vi "8.6-Crossbow Test.vi"() -> ()   [LabVIEW 2010]
uses:
  <vilib>/Instr/_visa.llb/VISA Configure Serial Port (Instr).vi
panel:
  in  "Array of Data to Send":u8[](array[numeric]) format="%.0x"
  in  "Use Checksum":bool
  out "error out":errorcluster
  out "Bytes at Port":u32
  in  "Stop Program":bool
  in  "baud rate (9600)":u32=38400
  in  "data bits (8)":u16=8
  in  "stop bits (10: 1 bit)":u16(ring)=10 items=["1.0"=10, "1.5"=15, "2.0"=20]
  in  "parity (0:none)":enum16{"None", "Odd", "Even", "Mark", "Space"}(ring)
  in  "Reset Port":bool
  in  "End Test":bool
  in  "VISA resource name":refnum<visa-resource-name>
  in  "Send String":bool
  out "Serial Port Output":string
  in  "String to write":string
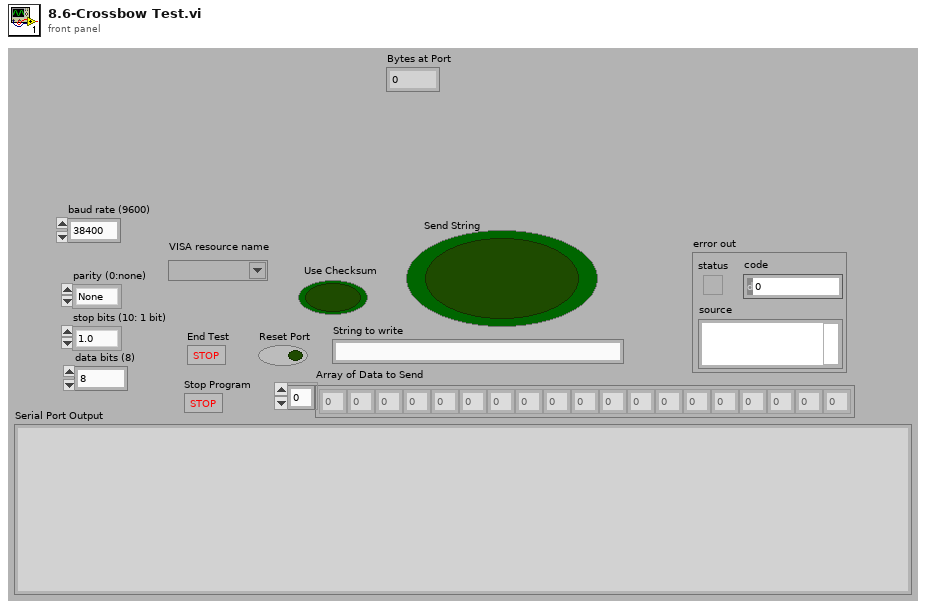
[diagram p1: front panel]
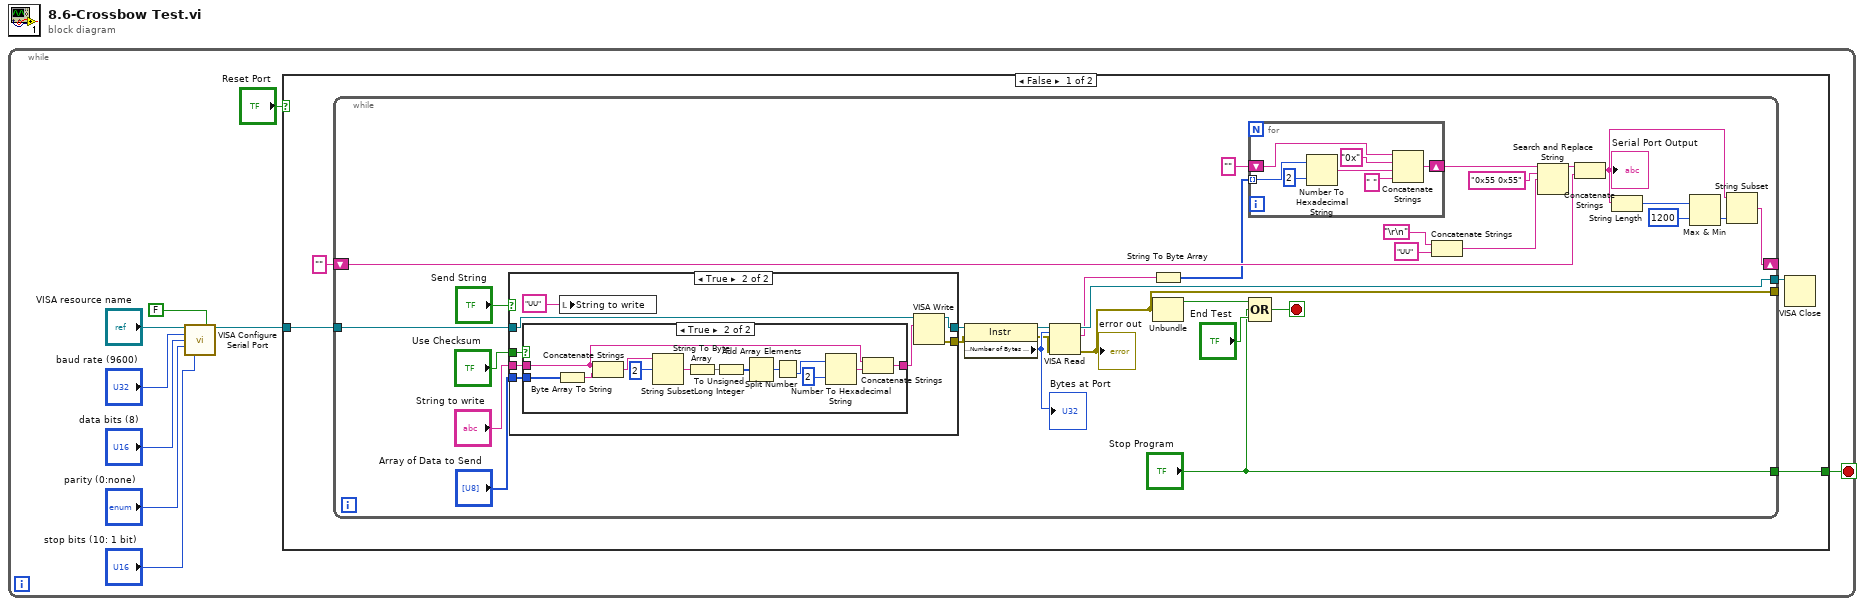
[diagram p0: block diagram]
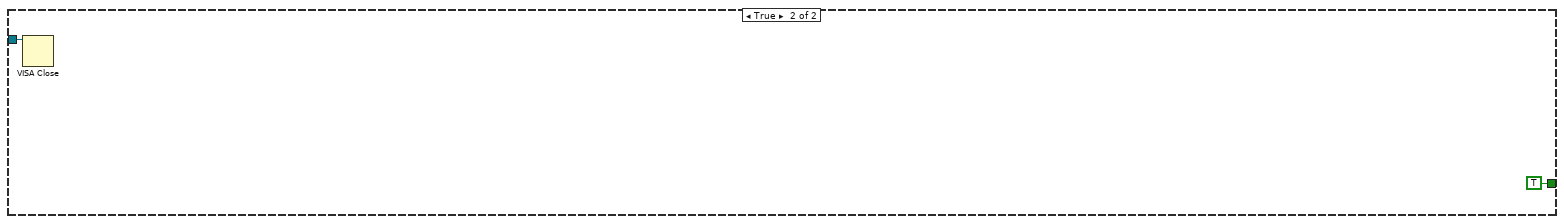
[diagram p4: hidden frame]
diagram:
  n1 = while {
    stop <- w1 stop-if-true
    n2 = call-poly "VISA Configure Serial Port"("VISA resource name"="VISA resource name", "Enable Termination\nChar (T)"=FALSE ("Enable Termination\nChar (T)"), "baud rate (9600)"="baud rate (9600)", "data bits (8)"="data bits (8)", "parity (0:none)"="parity (0:none)", "stop bits (10: 1 bit)"="stop bits (10: 1 bit)") -> ("VISA resource name out"=w8:refnum<visa-resource-name>)  [unwired: 8 in, 1 out]
    n3 = case shown="False" "Reset Port" {
      tunnel: w8 -> [w13 w76]
      tunnel: [w10 TRUE ("Stop Program")] -> w1
      frame False {
        n4 = while {
          tunnel: w13 -> [w44]
          tunnel: [w38] -> w12
          shift-right: [w36] -> _
          shift-left: "" ("String to write") -> [w25]
          tunnel: ["Stop Program"] -> w10
          tunnel: [w16] -> _
          stop <- w31 stop-if-true
          n5 = case shown="True" "Send String" {
            tunnel: w44 -> [w52 w60]
            tunnel: "String to write" -> [_ w55]
            tunnel: [w52 w58] -> w41
            tunnel: [_ w57] -> w28
            tunnel: "Use Checksum" -> [_ w56]
            tunnel: "Array of Data to Send" -> [_ w53]
            frame False {
            }
            frame True {
              n6 = case shown="True" w56 {
                tunnel: w55 -> [w61 w69]
                tunnel: [w61 w67] -> w54
                tunnel: w53 -> [_ w66]
                frame False {
                }
                frame True {
                  n7 = Byte Array To String(unsigned byte array=w66) -> (string=w64:string)
                  n8 = Concatenate Strings(w69, w64) -> (w65:string)
                  n9 = String Subset(string=w65, offset (0)=2) -> (substring=w73:string)  [unwired: 1 in]
                  n10 = String To Byte Array(string=w73) -> (unsigned byte array=w74:u8[])
                  n11 = To Unsigned Long Integer(number=w74) -> (unsigned 32bit integer=w71:u32[])
                  n12 = Add Array Elements(numeric array=w71) -> (sum=w63:u32)
                  n13 = Split Number(x=w63) -> (lo(x)=w62:u16)  [unwired: 1 out]
                  n14 = Number To Hexadecimal String(1:i16 2 ("width (-)"), 2:w62) -> (0:w68:string)
                  n15 = Concatenate Strings(w69, w68) -> (w67:string)
                }
              }
              n16 = local write "String to write"("UU" ("String to write")) -> ()
              n17 = VISA Write(VISA resource name=w60, write buffer=w54) -> (VISA resource name out=w58:refnum<visa-resource-name>, error out=w57:errorcluster)  [unwired: 1 in, 1 out]
            }
          }
          n18 = property class="Instr"(reference=w41, error in=w28) -> (reference out=w40:refnum<visa-resource-name>, error out=w29:errorcluster, "Serial Settings:Number of Bytes at Serial Port"=w39:u32)
          "Bytes at Port" <- w39
          n19 = VISA Read(VISA resource name=w40, byte count=w39, error in (no error)=w29) -> (VISA resource name out=w38:refnum<visa-resource-name>, read buffer=w20:string, error out=w16:errorcluster)  [unwired: 1 out]
          "error out" <- w16
          n20 = String To Byte Array(string=w20) -> (unsigned byte array=w18:u8[])
          n21 = Unbundle(w16) -> ("status"=w27:bool)  [unwired: 2 out]
          n22 = for {
            shift-right: [w45] -> w17
            shift-left: "" ("search string") -> [w46]
            tunnel: w18 -> [w51] mode=indexing
            n23 = Number To Hexadecimal String(1:i16 2 ("width (-)"), 2:w51) -> (0:w49:string)
            n24 = Concatenate Strings(w46, "0x", w49, " " ("string")) -> (w45:string)
          }
          n25 = Compound Arithmetic op=OR(w27, "Stop Program", "End Test") -> (w31:bool)
          n26 = Concatenate Strings("\r\n", "UU" ("search string")) -> (w22:string)
          n27 = Search and Replace String(input string=w17, search string="0x55 0x55", replace string=w22) -> (result string=w24:string)  [unwired: 5 in, 3 out]
          n28 = Concatenate Strings(w24, w25) -> (w37:string)
          "Serial Port Output" <- w37
          n29 = String Length(string=w37) -> (length=w35:i32)
          n30 = Max & Min(x=w35, y=1200) -> (min(x,y)=w34:i32)  [unwired: 1 out]
          n31 = String Subset(string=w37, length (rest)=w34) -> (substring=w36:string)  [unwired: 1 in]
        }
        n32 = VISA Close(VISA resource name=w12) -> ()  [unwired: 1 in, 1 out]
      }
      frame True {
        n33 = VISA Close(VISA resource name=w76) -> ()  [unwired: 1 in, 1 out]
      }
    }
  }
